vi "Set Relative Target Position.vi"(0 "reference in":refnum<class "SmartMotor.lvclass">, 2 "Relative Target Position (Revolutions)":dbl, 4 "Rotation Direction":u16(ring) items=["CW", "CCW"], 5 "error in (no error)":errorcluster) -> (14 "reference out":refnum<class "SmartMotor.lvclass">, 19 "error out":errorcluster)   [LabVIEW 2017, in "SmartMotor.lvclass"]
uses:
  SmartMotor.lvclass
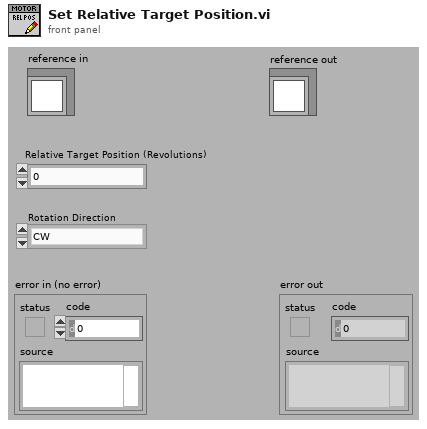
[diagram p1: front panel]
types:
  T1 = typedef "SmartMotor.lvclass/ObjectAttributes.ctl" = cluster{"SmartMotor Chain VISA Resource":refnum<visa-resource-name>, "SmartMotor Chain Address":i16, "Motor Absolute Position":i32, "Motor Relative Position":i32, "Motor Torque":i32, "Motor Voltage":i32, "Screwdriver Engaged":bool, "Screwdriver Torque Limit":i32, "Torque Monitor On/Off Status":bool, "Torque Monitor VI Reference":refnum<vi>, "Absolute Motor Torque (Filtered)":dbl, "SmartMotor Status":T2, "SmartMotor Error":T3}
  T2 = typedef "SmartMotor.lvclass/SmartMotor Status.ctl" = enum8{"Stopped", "Moving"}
  T3 = typedef "SmartMotor.lvclass/SmartMotor Error.ctl" = enum8{"None", "Read Error", "Low Voltage"}
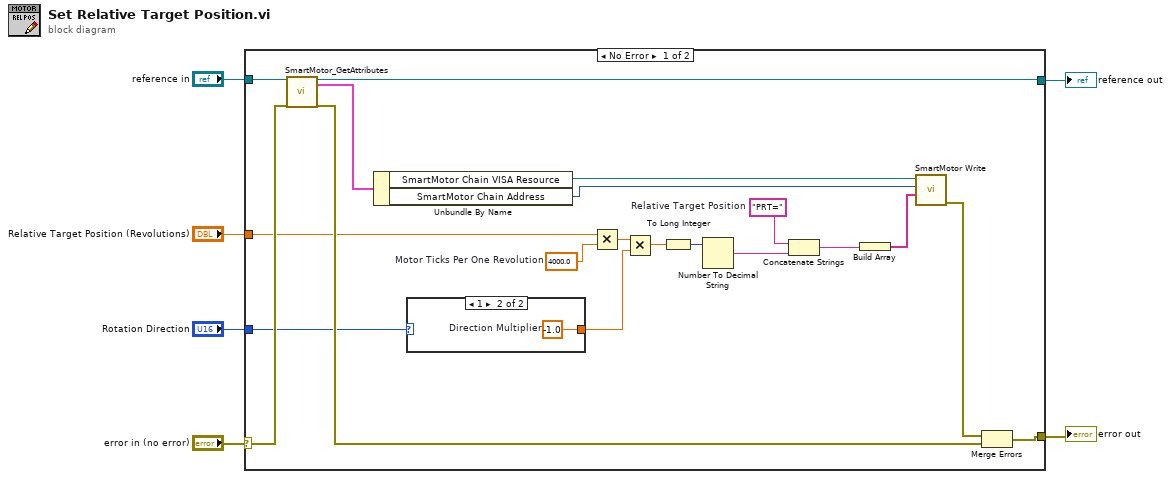
[diagram p0: block diagram]
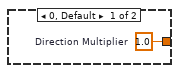
[diagram p2: hidden frame]
diagram:
  n1 = case shown="No Error" "error in (no error)" {
    selector: "error in (no error)" -> [w25 w30]
    tunnel: [w23 w30] -> w5
    tunnel: [w24 w29] -> w3
    tunnel: "reference in" -> [w26 w29]
    tunnel: "Relative Target Position (Revolutions)" -> [w20 _]
    tunnel: "Rotation Direction" -> [w19 _]
    frame No Error {
      w13 = "PRT="  # Relative Target Position
      w16 = 4000.0  # Motor Ticks Per One Revolution
      n2 = call "SmartMotor_GetAttributes.vi"("reference in"=w26, "error in (no error)"=w25) -> ("reference out"=w24:refnum<class "SmartMotor.lvclass">, "Data"=w7:T1, "error out"=w22:errorcluster)  [unwired: 14 in, 1 out]
      n3 = Unbundle By Name(w7) -> ("SmartMotor Chain VISA Resource"=w18:refnum<visa-resource-name>, "SmartMotor Chain Address"=w8:i16)
      n4 = case shown="1" w19 {
        tunnel: [w27 w28] -> w14
        frame 0, Default {
          w27 = 1.0  # Direction Multiplier
        }
        frame 1 {
          w28 = -1.0  # Direction Multiplier
        }
      }
      n5 = Multiply(x=w20, y=w16) -> (x*y=w15:dbl)
      n6 = Multiply(x=w15, y=w14) -> (x*y=w9:dbl)
      n7 = To Long Integer(number=w9) -> (32bit integer=w10:i32)
      n8 = Number To Decimal String(number=w10) -> (decimal integer string=w12:string)  [unwired: 1 in]
      n9 = Concatenate Strings(w13, w12) -> (w11:string)
      n10 = Build Array(w11) -> (w17:string[])
      n11 = call "SmartMotor Write.vi"("VISA resource IN"=w18, "Motor Number"=w8, "Motor Command Array"=w17) -> ("Error Out"=w21:errorcluster)  [unwired: 4 in, 2 out]
      n12 = Merge Errors(w21, w22) -> (w23:errorcluster)
    }
    frame Error {
    }
  }
  "error out" <- w5
  "reference out" <- w3
